vi "PH_Beckhoff_PPMA-Rods.ProcPeriodic.vi"(0 "i ref in":refnum<vi>, 3 "ms timeout (10000)":i32=10000, 5 "error in (no error)":errorcluster) -> (14 "i ref out":refnum<vi>, 17 "timed out":bool, 19 "error out":errorcluster)   [LabVIEW 2014, in "PH_Beckhoff_PPMA-Rods.lvlib"]
doc: "This method serves to periodically do things like reading values from the HW. Methods that should be executed periodically should be called from THIS methode. Add code here."
uses:
  PH_Beckhoff_PPMA-Rods.lvlib
  PH_Beckhoff/PH_Beckhoff.lvlib
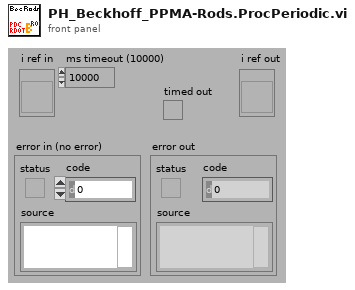
[diagram p1: front panel]
types:
  T1 = typedef "PH_Beckhoff.lvlib/PH_Beckhoff.i attribute.ctl" = cluster{"GUI Refs":T2, "operation?":bool, "Default Prdc Interval":i32, "Connection":T3, "AMS Net ID":T4, "Klemmencluster: # of":T5, "Values":T6, "IP":string, "Description":string, "configured?":bool, "Change Manager":cluster{"Detemination wanted?":bool, "Values changed at":cluster{"Sonderklemmen Inputs":i32[], "Analog Inputs":i32[], "Analog Outputs":i32[], "Digital Inputs":i32[], "Digital Outputs":i32[]}}, "Difference to handle an analog input as change":u32}
  T2 = typedef "PH_Beckhoff.lvlib/PH_Beckhoff.GUI Refs.ctl" = cluster{"ADS Error":refnum<vi>, "Values":refnum<vi>, "configured?":refnum<vi>, "Connection":refnum<vi>, "IP":refnum<vi>, "Prdc Int [ms]":refnum<vi>}
  T3 = typedef "PH_Beckhoff.lvlib/PH_Beckhoff.Connectivity.ctl" = cluster{"DLL?":bool, "Port?":bool, "Client?":bool, "Ping?":bool, "unsuccessful Pings":u32}
  T4 = typedef "Beckhoff - Driver np.lvlib/Beckhoff Access.ctl" = cluster{"DLL path":path, "AMS Net ID":cluster{"1st # of IP":u8, "2nd # of IP":u8, "3rd # of IP":u8, "4th # of IP":u8, "In Port":u8, "Out Port":u8}}
  T5 = typedef "Beckhoff - Driver np.lvlib/Klemmendeclarer.ctl" = cluster{"Offset due to Sonderklemms":u32, "analog Inputs":u32, "analog Outputs":u32, "digital Input Bits":u32, "digital Output Bits":u32}
  T6 = typedef "PH_Beckhoff.lvlib/PH_Beckhoff.Values.ctl" = cluster{"Sonderklemmen Inputs":T7, "Analog Inputs":T8, "Analog Outputs":T10, "Digital Inputs":T11, "Digital Outputs":T12}
  T7 = typedef "PH_Beckhoff.lvlib/PH_Beckhoff.Sonderklemmen Inputs.ctl" = cluster{"Total Length":u32, "Name":string, "Value":u64, "Quality":bool, "Service ID":i32, "Offset":u32, "Length":u32}[]
  T8 = typedef "PH_Beckhoff.lvlib/PH_Beckhoff.Analog Inputs.ctl" = cluster{"Name":string, "Value":u32, "Quality":bool, "Service ID":i32, "Sca Type":T9}[]
  T9 = typedef "PH_Beckhoff.lvlib/PH_Beckhoff.Scaling Type.ctl" = enum16{"none", "0 ... 15 Bit -> 0 ... 5", "0 ... 15 Bit -> 0 ... 10", "0 ... 15 Bit -> 0 ... 25", "0 ... 15 Bit -> 4 ... 20", "0 ... 15 Bit -> 0 ... 1", "0 ... 15 Bit -> 0 ... 20000", "0 ... 15 Bit -> 0 ... 24000"}
  T10 = typedef "PH_Beckhoff.lvlib/PH_Beckhoff.Analog Outputs.ctl" = cluster{"Name":string, "Value":u32, "Quality":bool, "Wanted Value":u32, "Service ID":i32, "Sca Type":T9}[]
  T11 = typedef "PH_Beckhoff.lvlib/PH_Beckhoff.Digital Inputs.ctl" = cluster{"Name":string, "Value":bool, "Quality":bool, "Service ID":i32, "inverted?":bool}[]
  T12 = typedef "PH_Beckhoff.lvlib/PH_Beckhoff.Digital Outputs.ctl" = cluster{"Name":string, "Value":bool, "Quality":bool, "Wanted Value":bool, "Service ID":i32, "inverted?":bool}[]
  T13 = typedef "PH_Beckhoff_PPMA-Rods.lvlib/PH_Beckhoff_PPMA-Rods.i attribute.ctl" = cluster{"Input Up GUI Refs":refnum<vi>[], "Output GUI Refs":cluster{"Rod A up":refnum<vi>, "Rod B up":refnum<vi>, "Warnlamp orange":refnum<vi>, "Warnlamp green":refnum<vi>}, "States":cluster{"GUI Ref":refnum<vi>, "Status":T14, "Service ID":i32}[], "Input GUI Refs":cluster{"earth ok":refnum<vi>, "door locked K1":refnum<vi>, "door locked K2":refnum<vi>, "valve closed":refnum<vi>}}
  T14 = typedef "PH_StatusHandler.lvlib/PH_StatusHandler.Status.ctl" = i16
  T15 = cluster{"GUI Ref":refnum<vi>, "Status":T14, "Service ID":i32}[]
  T16 = cluster{"earth ok":refnum<vi>, "door locked K1":refnum<vi>, "door locked K2":refnum<vi>, "valve closed":refnum<vi>}
  T17 = cluster{"Rod A up":refnum<vi>, "Rod B up":refnum<vi>, "Warnlamp orange":refnum<vi>, "Warnlamp green":refnum<vi>}
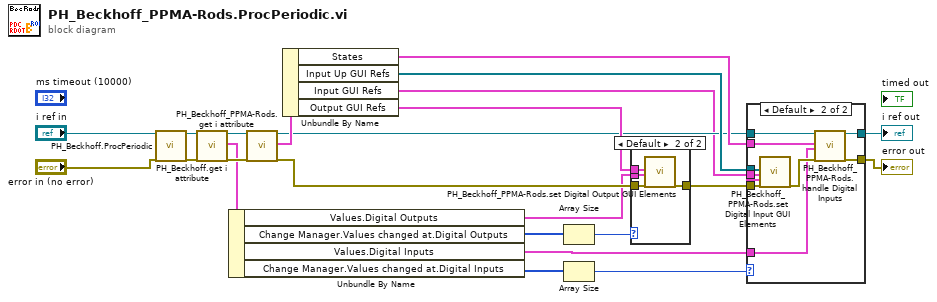
[diagram p0: block diagram]
diagram:
  n1 = call "PH_Beckhoff.ProcPeriodic.vi"("i ref in"="i ref in", "error in (no error)"="error in (no error)") -> ("i ref out"=w19:refnum<vi>, "error out"=w21:errorcluster)  [unwired: 15 in, 1 out]
  n2 = call "PH_Beckhoff.get i attribute.vi"("i ref in"=w19, "error in (no error)"=w21) -> ("i ref out"=w18:refnum<vi>, "i attribute"=w17:T1, "error out"=w20:errorcluster)  [unwired: 15 in]
  n3 = Unbundle By Name(w17) -> ("Values.Digital Outputs"=w13:T12, "Change Manager.Values changed at.Digital Outputs"=w4:i32[], "Values.Digital Inputs"=w6:T11, "Change Manager.Values changed at.Digital Inputs"=w3:i32[])
  n4 = call "PH_Beckhoff_PPMA-Rods.get i attribute.vi"("i ref in"=w18, "error in (no error)"=w20) -> ("i ref out"=w8:refnum<vi>, "i attribute"=w16:T13, "error out"=w14:errorcluster)  [unwired: 15 in]
  n5 = Unbundle By Name(w16) -> ("States"=w9:T15, "Input Up GUI Refs"=w11:refnum<vi>[], "Input GUI Refs"=w5:T16, "Output GUI Refs"=w12:T17)
  n6 = Array Size(array=w4) -> (size(s)=w2:i32)
  n7 = Array Size(array=w3) -> (size(s)=w1:i32)
  n8 = case shown="Default" w2 {
    tunnel: [w24 w28] -> w15
    tunnel: w14 -> [w24 w27]
    tunnel: w13 -> [_ w26]
    tunnel: w12 -> [_ w25]
    frame 0 {
    }
    frame Default {
      n9 = call "PH_Beckhoff_PPMA-Rods.set Digital Output GUI Elements.vi"("Output GUI Refs"=w25, "Digital Outputs"=w26, "error in"=w27) -> ("error out"=w28:errorcluster)  [unwired: 16 in]
    }
  }
  n10 = case shown="Default" w1 {
    tunnel: w15 -> [w29 w39]
    tunnel: w11 -> [_ w37]
    tunnel: [w29 w36] -> w10
    tunnel: w9 -> [_ w31]
    tunnel: w8 -> [w30 w35]
    tunnel: [w30 w34] -> w7
    tunnel: w6 -> [_ w33]
    tunnel: w5 -> [_ w32]
    frame 0 {
    }
    frame Default {
      n11 = call "PH_Beckhoff_PPMA-Rods.set Digital Input GUI Elements.vi"("Input Up GUI Refs"=w37, "Input GUI Refs"=w32, "Digital Inputs"=w33, "error in"=w39) -> ("error out"=w38:errorcluster)  [unwired: 15 in]
      n12 = call "PH_Beckhoff_PPMA-Rods.handle Digital Inputs.vi"("i ref in"=w35, "States"=w31, "Digital Inputs"=w33, "error in"=w38) -> ("i ref out"=w34:refnum<vi>, "error out"=w36:errorcluster)  [unwired: 14 in]
    }
  }
  "error out" <- w10
  "i ref out" <- w7
